vi "Sort STEPs.vi"(8 "error in (no error)":errorcluster, 11 "All Sequence STEPs in":refnum<class "STEP.lvclass">[](array[class])) -> (0 "error out":errorcluster, 3 "All Sequence STEPs":refnum<class "STEP.lvclass">[](array[class]))   [LabVIEW 2014, in "SeqLoop.lvlib"]
uses:
  SeqLoop.lvlib
  Classes/STEP/STEP.lvclass
  Classes/STEP/STEP.lvclass/STEP.ctl
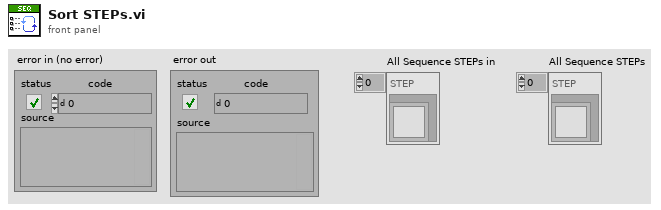
[diagram p1: front panel]
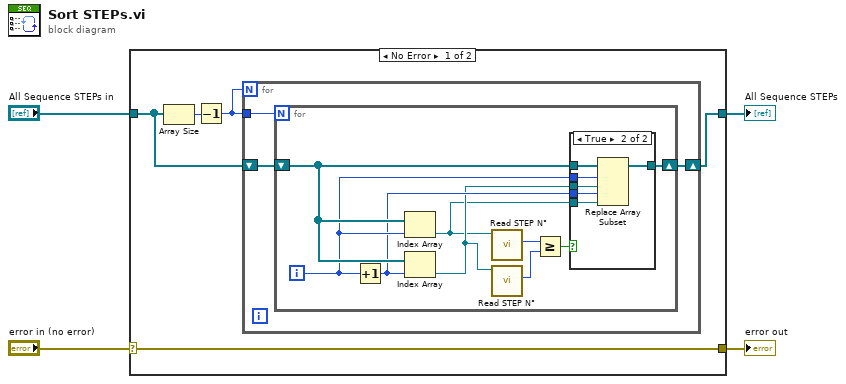
[diagram p0: block diagram]
diagram:
  n1 = case shown="No Error" "error in (no error)" {
    selector: "error in (no error)" -> [w5 w29]
    tunnel: "All Sequence STEPs in" -> [w7 w30]
    tunnel: [w6 w30] -> w3
    tunnel: [w5 w29] -> w2
    frame No Error {
      n2 = Array Size(array=w7) -> (size(s)=w9:i32)
      n3 = Decrement(x=w9) -> (x-1=w8:i32)
      n4 = for {
        N: w8 -> [_]
        shift-right: [w11] -> w6
        shift-left: w7 -> [w12]
        tunnel: w8 -> [w10]
        n5 = for {
          N: w10 -> [_]
          shift-right: [w20] -> w11
          shift-left: w12 -> [w19]
          i -> [w18]
          n6 = Increment(x=w18) -> (x+1=w17:i32)
          n7 = Index Array(array=w19, index=w18) -> (element=w14:refnum<class "STEP.lvclass">)
          n8 = Index Array(array=w19, index=w17) -> (element=w16:refnum<class "STEP.lvclass">)
          n9 = call "Read STEP N°.vi"("STEP in"=w14) -> ("STEP N°"=w13:u32)  [unwired: 9 in, 1 out]
          n10 = call "Read STEP N°.vi"("STEP in"=w16) -> ("STEP N°"=w15:u32)  [unwired: 9 in, 1 out]
          n11 = Greater Or Equal?(x=w13, y=w15) -> (x >= y?=w21:bool)
          n12 = case shown="True" w21 {
            tunnel: [w22 w28] -> w20
            tunnel: w19 -> [w22 w27]
            tunnel: w14 -> [_ w26]
            tunnel: w16 -> [_ w25]
            tunnel: w18 -> [_ w24]
            tunnel: w17 -> [_ w23]
            frame False {
            }
            frame True {
              n13 = Replace Array Subset(array=w27, new element #1=w25, index #1=w24, new element #2=w26, index #2=w23) -> (w28:refnum<class "STEP.lvclass">[])
            }
          }
        }
      }
    }
    frame Error {
    }
  }
  "error out" <- w2
  "All Sequence STEPs" <- w3
